vi "Test.vi"() -> ()   [LabVIEW 2015]
uses:
  IRB/x86_32/IRB.lvlib
panel:
  in  "state":u32(ring) items=["IRB_RELAY_STATE_OFF", "IRB_RELAY_STATE_ON"]
  in  "index":u32
  out "Power 8":cluster{"voltage":dbl, "current":dbl}
  out "Power 7":cluster{"voltage":dbl, "current":dbl}
  out "Power 6":cluster{"voltage":dbl, "current":dbl}
  out "Power 5":cluster{"voltage":dbl, "current":dbl}
  out "Power 4":cluster{"voltage":dbl, "current":dbl}
  out "Power 3":cluster{"voltage":dbl, "current":dbl}
  out "Power 2":cluster{"voltage":dbl, "current":dbl}
  out "Power 1":cluster{"voltage":dbl, "current":dbl}
  out "Power 0":cluster{"voltage":dbl, "current":dbl}
  out "State Mask":u16 format="%016b"
  out "Fault Mask":u16 format="%016b"
  in  "New State Mask":u16 format="%016b"
  out "error out":errorcluster caption="Fehler (Ausgang)"
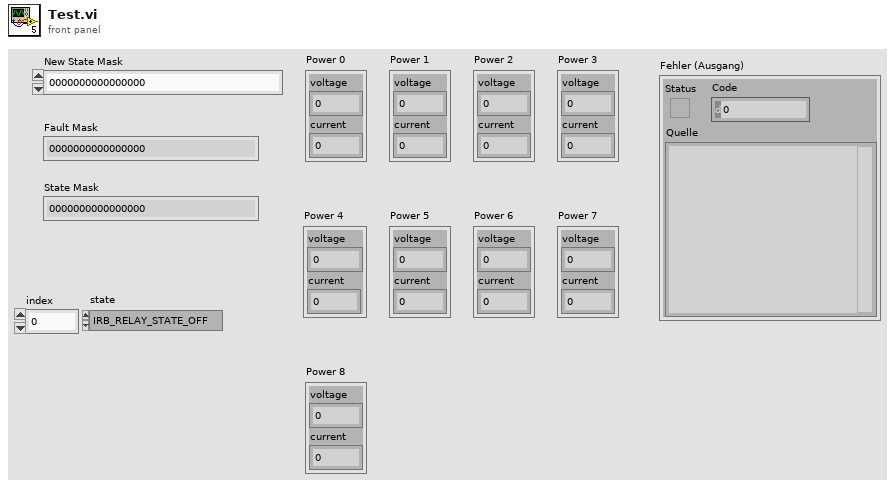
[diagram p1: front panel]
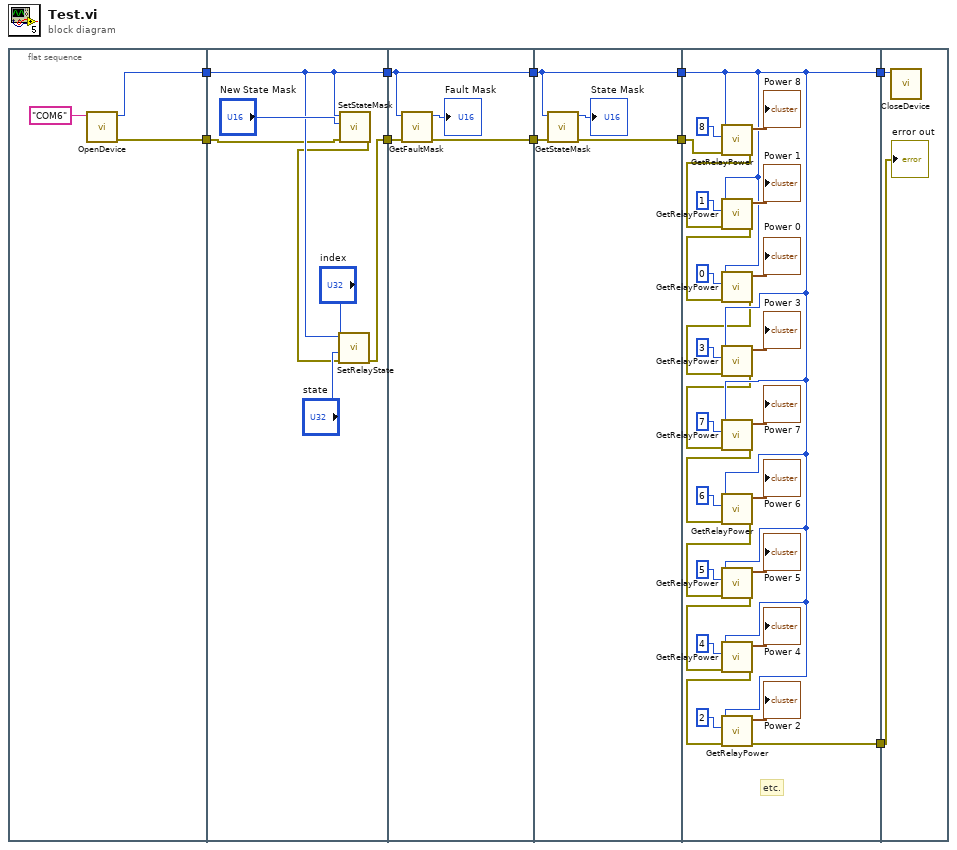
[diagram p0: block diagram]
diagram:
  n1 = flat-sequence {
    tunnel: [w12] -> w10
    tunnel: [w11] -> w8
    tunnel: w10 -> [w15]
    tunnel: [w16] -> w9
    tunnel: w8 -> [w19]
    tunnel: [w19] -> w4
    tunnel: w9 -> [w24]
    tunnel: [w23] -> w7
    tunnel: [w21] -> w6
    tunnel: w4 -> [w21]
    tunnel: w7 -> [w28]
    tunnel: w6 -> [w26]
    tunnel: [w26] -> w5
    tunnel: [w25] -> w3
    tunnel: w5 -> [w38]
    tunnel: w3 -> [w39]
    tunnel: [w38] -> w2
    tunnel: [w29] -> w1
    tunnel: w2 -> [w59]
    tunnel: w1 -> [w58]
    frame #0 {
      n2 = call "OpenDevice.vi"("port"="COM6") -> ("error out"=w12:errorcluster, "device"=w11:u32)  [unwired: 8 in, 1 out]
    }
    frame #1 {
      n3 = call "SetStateMask.vi"("error in (no error)"=w15, "mask"="New State Mask", "device"=w19) -> ("error out"=w14:errorcluster)  [unwired: 7 in, 1 out]
      n4 = call "SetRelayState.vi"("error in (no error)"=w14, "state"="state", "index"="index", "device"=w19) -> ("error out"=w16:errorcluster)  [unwired: 6 in, 1 out]
    }
    frame #2 {
      n5 = call "GetFaultMask.vi"("error in (no error)"=w24, "device"=w21) -> ("error out"=w23:errorcluster, "mask"=→"Fault Mask":u16)  [unwired: 7 in, 1 out]
    }
    frame #3 {
      n6 = call "GetStateMask.vi"("error in (no error)"=w28, "device"=w26) -> ("error out"=w25:errorcluster, "mask"=→"State Mask":u16)  [unwired: 7 in, 1 out]
    }
    frame #4 {
      # "etc."
      n7 = call "GetRelayPower.vi"("error in (no error)"=w39, "index"=u32 8, "device"=w38) -> ("error out"=w37:errorcluster, "power"=→"Power 8":cluster{"voltage":dbl, "current":dbl})  [unwired: 6 in, 1 out]
      n8 = call "GetRelayPower.vi"("error in (no error)"=w37, "index"=u32 1, "device"=w38) -> ("error out"=w36:errorcluster, "power"=→"Power 1":cluster{"voltage":dbl, "current":dbl})  [unwired: 6 in, 1 out]
      n9 = call "GetRelayPower.vi"("error in (no error)"=w36, "index"=u32 0, "device"=w38) -> ("error out"=w35:errorcluster, "power"=→"Power 0":cluster{"voltage":dbl, "current":dbl})  [unwired: 6 in, 1 out]
      n10 = call "GetRelayPower.vi"("error in (no error)"=w35, "index"=u32 3, "device"=w38) -> ("error out"=w34:errorcluster, "power"=→"Power 3":cluster{"voltage":dbl, "current":dbl})  [unwired: 6 in, 1 out]
      n11 = call "GetRelayPower.vi"("error in (no error)"=w34, "index"=u32 7, "device"=w38) -> ("error out"=w33:errorcluster, "power"=→"Power 7":cluster{"voltage":dbl, "current":dbl})  [unwired: 6 in, 1 out]
      n12 = call "GetRelayPower.vi"("error in (no error)"=w33, "index"=u32 6, "device"=w38) -> ("error out"=w32:errorcluster, "power"=→"Power 6":cluster{"voltage":dbl, "current":dbl})  [unwired: 6 in, 1 out]
      n13 = call "GetRelayPower.vi"("error in (no error)"=w32, "index"=u32 5, "device"=w38) -> ("error out"=w31:errorcluster, "power"=→"Power 5":cluster{"voltage":dbl, "current":dbl})  [unwired: 6 in, 1 out]
      n14 = call "GetRelayPower.vi"("error in (no error)"=w31, "index"=u32 4, "device"=w38) -> ("error out"=w30:errorcluster, "power"=→"Power 4":cluster{"voltage":dbl, "current":dbl})  [unwired: 6 in, 1 out]
      n15 = call "GetRelayPower.vi"("error in (no error)"=w30, "index"=u32 2, "device"=w38) -> ("error out"=w29:errorcluster, "power"=→"Power 2":cluster{"voltage":dbl, "current":dbl})  [unwired: 6 in, 1 out]
    }
    frame #5 {
      n16 = call "CloseDevice.vi"("device"=w59) -> ()  [unwired: 9 in, 2 out]
      "error out" <- w58
    }
  }
